vi "Close Pump.vi"(7 "Pump ID (0:A)":T1, 8 "error in (no error)":errorcluster, 11 "VISA resource in":refnum<visa-resource-name>) -> (0 "error out":errorcluster, 3 "VISA resource out":refnum<visa-resource-name>)   [LabVIEW 2020, in "Global FIA milliGAT.lvlib"]
doc: "Performs an instrument error query before terminating the software connection to the instrument."
uses:
  <instrlib>/RxnRover/Global FIA milliGAT 3.14/Global FIA milliGAT.lvlib
  <instrlib>/RxnRover/Global FIA milliGAT 3.14/Public/Utility/Pump Address.ctl
  <instrlib>/RxnRover/Global FIA milliGAT 3.14/Private/Pump Parameter.ctl
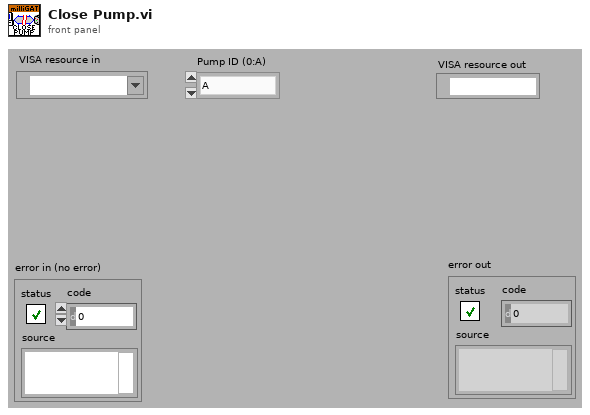
[diagram p1: front panel]
types:
  T1 = typedef "Global FIA milliGAT.lvlib/Pump Address.ctl" = enum16{"A", "B", "C", "D", "E", "F", "G", "H", "I", "J", "K", "L", "M", "N", "O", "P", "Q", "R", "S", "T", "U", "V", "W", "X", "Y", "Z", "a", "b", "c", "d", "e", "f", "g", "h", "i", "j", "k", "l", "m", "n", "o", "p", "q", "r", "s", "t", "u", "v", "w", "x", "y", "z", "0", "1", "2", "3", "4", "5", "6", "7", "8", "9"}
  T2 = typedef "Global FIA milliGAT.lvlib/Pump Parameter.ctl" = enum16{"Enabled", "EU", "EU Calibration Factor", "Fixed Asp or Disp", "Starting Position", "Starting Flow", "Peak Flow", "Flow Acceleration", "Flow Deceleration", "Session Volume", "Max Pressure", "Backlash (usteps)", "BL Calibration Factor", "BL Correction Enabled", "Min Flow", "Max Flow", "Min Acceleration", "Max Acceleration", "Service Volume", "Life Volume"}
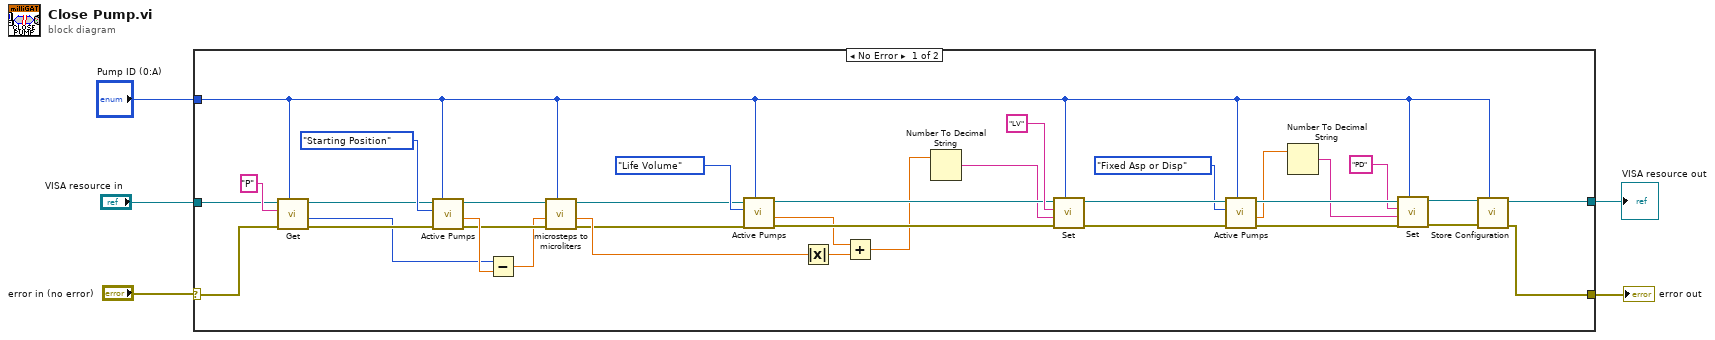
[diagram p0: block diagram]
diagram:
  n1 = case shown="No Error" "error in (no error)" {
    selector: "error in (no error)" -> [w8 w42]
    tunnel: "Pump ID (0:A)" -> [w10 _]
    tunnel: "VISA resource in" -> [w9 w41]
    tunnel: [w7 w42] -> w3
    tunnel: [w6 w41] -> w2
    frame No Error {
      n2 = call <instrlib>:"Get.vi"("Pump ID (0:A)"=w10, "error in (no error)"=w8, "Parameter"="P" ("Parameter or Flag"), "VISA resource in"=w9) -> ("error out"=w20:errorcluster, "Value"=w17:i32, "VISA resource out"=w21:refnum<visa-resource-name>)  [unwired: 5 in]
      n3 = call <instrlib>:"Active Pumps.vi"("Pump ID (0:A)"=w10, "error in (no error)"=w20, "Parameter"=Pump_Parameter."Starting Position", "VISA resource in"=w21) -> ("error out"=w24:errorcluster, "Value out"=w25:dbl, "VISA resource out"=w23:refnum<visa-resource-name>)  [unwired: 4 in, 1 out]
      n4 = Subtract(x=w17, y=w25) -> (x-y=w18:dbl)
      n5 = call <instrlib>:"microsteps to microliters.vi"("Pump ID (0:A)"=w10, "error in (no error)"=w24, "Microsteps (0)"=w18, "VISA resource in"=w23) -> ("error out"=w15:errorcluster, "Microliters"=w19:dbl, "VISA resource out"=w16:refnum<visa-resource-name>)  [unwired: 5 in]
      n6 = call <instrlib>:"Active Pumps.vi"("Pump ID (0:A)"=w10, "error in (no error)"=w15, "Parameter"=Pump_Parameter."Life Volume", "VISA resource in"=w16) -> ("error out"=w37:errorcluster, "Value out"=w13:dbl, "VISA resource out"=w38:refnum<visa-resource-name>)  [unwired: 4 in, 1 out]
      n7 = Absolute Value(x=w19) -> (abs(x)=w14:dbl)
      n8 = Add(x=w13, y=w14) -> (x+y=w12:dbl)
      n9 = Number To Decimal String(number=w12) -> (decimal integer string=w11:string)  [unwired: 1 in]
      n10 = call <instrlib>:"Set.vi"("Pump ID (0:A)"=w10, "error in (no error)"=w37, "Expression"=w11, "Parameter"="LV" ("Parameter Name"), "VISA resource in"=w38) -> ("error out"=w35:errorcluster, "VISA resource out"=w36:refnum<visa-resource-name>)  [unwired: 5 in]
      n11 = call <instrlib>:"Active Pumps.vi"("Pump ID (0:A)"=w10, "error in (no error)"=w35, "Parameter"=Pump_Parameter."Fixed Asp or Disp", "VISA resource in"=w36) -> ("error out"=w29:errorcluster, "Value out"=w31:dbl, "VISA resource out"=w33:refnum<visa-resource-name>)  [unwired: 4 in, 1 out]
      n12 = Number To Decimal String(number=w31) -> (decimal integer string=w30:string)  [unwired: 1 in]
      n13 = call <instrlib>:"Set.vi"("Pump ID (0:A)"=w10, "error in (no error)"=w29, "Expression"=w30, "Parameter"="PD", "VISA resource in"=w33) -> ("error out"=w27:errorcluster, "VISA resource out"=w28:refnum<visa-resource-name>)  [unwired: 5 in]
      n14 = call <instrlib>:"Store Configuration.vi"("Pump ID (0:A)"=w10, "error in (no error)"=w27, "VISA resource in"=w28) -> ("error out"=w7:errorcluster, "VISA resource out"=w6:refnum<visa-resource-name>)  [unwired: 7 in]
    }
    frame Error {
    }
  }
  "error out" <- w3
  "VISA resource out" <- w2
